vi "Init Loop Data.vi"(7 "TX Q":refnum<queue>, 11 "RemoteDataService in":refnum<class "RemoteDataService.lvclass">) -> (0 "error out":errorcluster, 3 "Loop Data":T1)   [LabVIEW 2020, in "Vecto.lvlib" / "RemoteDataService.lvclass"]
uses:
  RemoteDataService.lvclass
  Loop Data.ctl
  SequenceCountService/SequenceCountService.lvclass
  ChannelService/ChannelService.lvclass
  Published Group.ctl
  Packet.ctl
  lv-protoc/LV-Proto/Message/Message.lvclass
  Group Data Type.ctl
  Subscription.ctl
  Subscription Info.ctl
  SubscribedDataHandler/SubscribedDataHandler.lvclass
  VectoConfig/Telemetry Config.ctl
  VectoConfig/Telemetry Routing.ctl
  VectoConfig/Endpoint.ctl
  RemoteDataService.lvclass/RemoteDataService.ctl
  Address Type.vi
  Resolve Address Type.vi
  Resolve Address Type.vi/f8bc95ce-8757-4bea-a9a5-74e77d021f7a.vi
  <vilib>/AdvancedString/1D String Array to Delimited String.vi
  <vilib>/Utility/error.llb/Error Cluster From Error Code.vi
  <vilib>/Comparison/Equal/Equal Functor/Equal Functor.lvclass
  VectoConfig/VectoConfig.lvlib
  IP Resolver/IP Resolver.lvclass
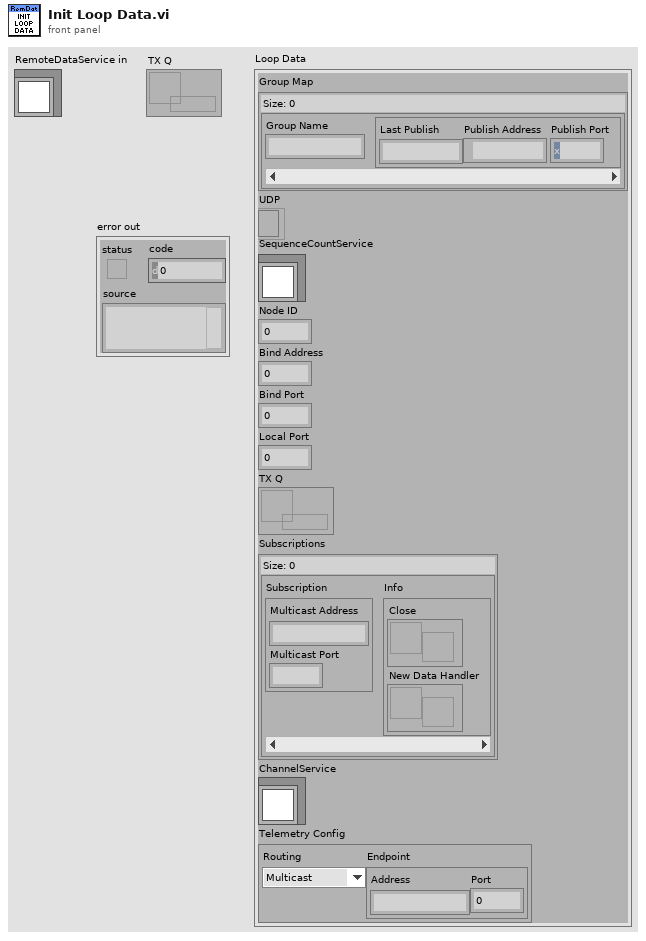
[diagram p1: front panel]
types:
  T1 = typedef "Vecto.lvlib/RemoteDataService.lvclass/Loop Data.ctl" = cluster{"Group Map":map{string, T2}, "UDP":refnum<k16>, "SequenceCountService":refnum<class "SequenceCountService.lvclass">, "Node ID":u32, "Bind Address":u32, "Bind Port":u16, "Local Port":u16, "TX Q":refnum<queue>, "Subscriptions":map{T3, T4}, "ChannelService":refnum<class "ChannelService.lvclass">, "Telemetry Config":T5}
  T2 = typedef "Vecto.lvlib/RemoteDataService.lvclass/Published Group.ctl" = cluster{"Last Publish":dbl, "Publish Address":u32, "Publish Port":u16}
  T3 = typedef "Vecto.lvlib/RemoteDataService.lvclass/Subscription.ctl" = cluster{"Multicast Address":string, "Multicast Port":u16}
  T4 = typedef "Vecto.lvlib/RemoteDataService.lvclass/Subscription Info.ctl" = cluster{"Close":refnum<user-event>, "New Data Handler":refnum<user-event>}
  T5 = typedef "VectoConfig.lvlib/Telemetry Config.ctl" = cluster{"Routing":T6, "Endpoint":T7}
  T6 = typedef "VectoConfig.lvlib/Telemetry Routing.ctl" = enum16{"Multicast", "Unicast"}
  T7 = typedef "VectoConfig.lvlib/Endpoint.ctl" = cluster{"Address":string, "Port":u16}
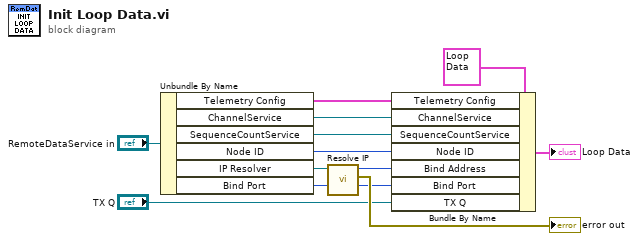
[diagram p0: block diagram]
diagram:
  n1 = Unbundle By Name("RemoteDataService in") -> ("Telemetry Config"=w3:T5, "ChannelService"=w4:refnum<class "ChannelService.lvclass">, "SequenceCountService"=w8:refnum<class "SequenceCountService.lvclass">, "Node ID"=w7:u32, "IP Resolver"=w2:refnum<class "IP Resolver.lvclass">, "Bind Port"=w6:u16)
  n2 = call "Resolve IP.vi"("IP Resolver in"=w2) -> ("error out"=→"error out":errorcluster, "U32 Address"=w1:u32)  [unwired: 9 in]
  n3 = Bundle By Name(cluster=T1 {"Group Map"={}, "UDP"=refnum, "SequenceCountService"=refnum, "Node ID"=0, "Bind Address"=0, "Bind Port"=0, "Local Port"=0, "TX Q"=refnum, "Subscriptions"={}, "ChannelService"=refnum, "Telemetry Config"={"Routing"=enum."Multicast", "Endpoint"={"Address"="", "Port"=0}}} ("Loop Data"), "Telemetry Config"=w3, "ChannelService"=w4, "SequenceCountService"=w8, "Node ID"=w7, "Bind Address"=w1, "Bind Port"=w6, "TX Q"="TX Q") -> (→"Loop Data":T1)
